vi "labview_results_get.vi"(0 "Path":path, 1 "Dust ID":string, 5 "Upper Timestamp":dbl, 7 "Velocity Limits":cluster{dbl, dbl}, 8 "Lower Timestamp":dbl, 11 "Min mass":dbl, 12 "Particle Quality":cluster{i32, i32}, 13 "Max mass":dbl, 14 "Session Quality":cluster{i32, i32}, 15 "Experiment ID":string, 16 "Make heatmap":bool, 17 "Dust Material":string) -> (20 "Results Output":string, 21 "Results Error/Debug":string, 25 "Request":string)   [LabVIEW 2015]
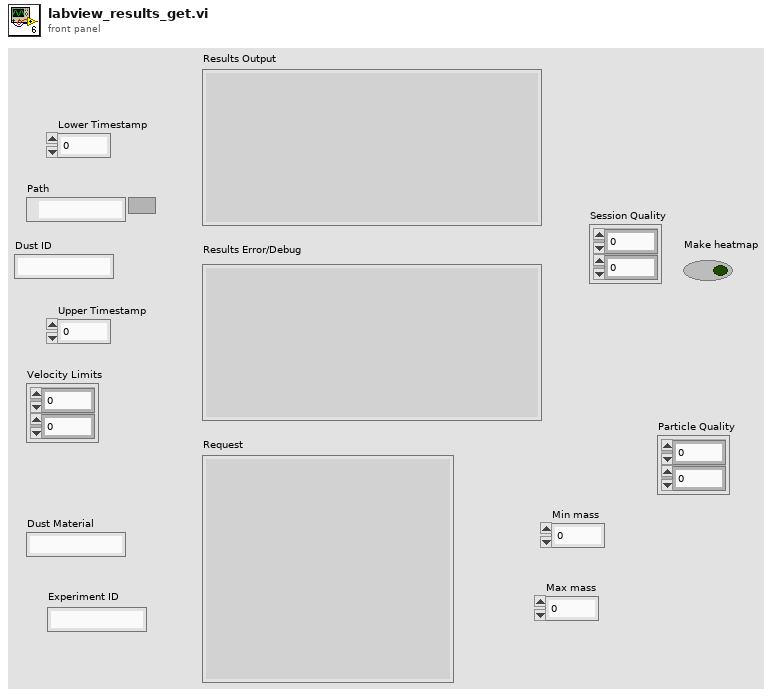
[diagram p1: front panel]
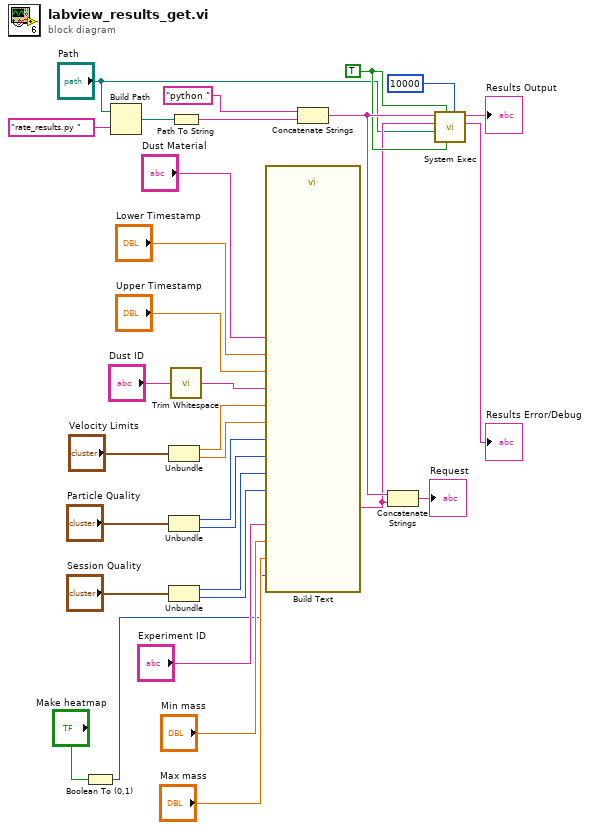
[diagram p0: block diagram]
diagram:
  w26 = TRUE
  n1 = Boolean To (0,1)(Boolean="Make heatmap") -> (0, 1=w1:i16)
  n2 = Build Path(base path="Path", name or relative path="rate_results.py ") -> (appended path=w8:path)
  n3 = Unbundle("Velocity Limits") -> (w20:dbl, w19:dbl)
  n4 = Unbundle("Particle Quality") -> (w14:i32, w13:i32)
  n5 = Unbundle("Session Quality") -> (w17:i32, w16:i32)
  n6 = Path To String(path=w8) -> (string=w7:string)
  n7 = call <vilib>:"Trim Whitespace.vi"("string"="Dust ID") -> ("trimmed string"=w22:string)  [unwired: 1 in]
  n8 = call "Build Text"("start"="Lower Timestamp", "stop"="Upper Timestamp", "dustID"=w22, "vmin"=w20, "vmax"=w19, "material"="Dust Material", "pq_min"=w14, "pq_max"=w13, "sq_min"=w17, "sq_max"=w16, "experiment_ID"="Experiment ID", "min_mass"="Min mass", "max_mass"="Max mass", "make_heatmap"=w1) -> ("Result"=w21:string)  [unwired: 12 in, 1 out]
  n9 = Concatenate Strings("python ", w7) -> (w30:string)
  n10 = Concatenate Strings(w30, w21) -> (→"Request":string)
  n11 = call <vilib>:"System Exec.vi"("expected output size  (4096)"=10000, "run minimized? (F)"=w26, "wait until completion? (T)"=w26, "working directory"="Path", "standard input"=w21, "command line"=w30) -> ("standard error"=→"Results Error/Debug":string, "standard output"=→"Results Output":string)  [unwired: 2 in, 2 out]
